vi "KM101_SetChannelZero.vi"(9 "Channel":i32, 10 "reference in":refnum<k7>) -> (2 "reference out":refnum<k7>)   [LabVIEW 2018, in "KIM101lib.lvlib"]
uses:
  KIM101lib.lvlib
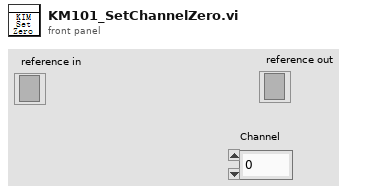
[diagram p1: front panel]
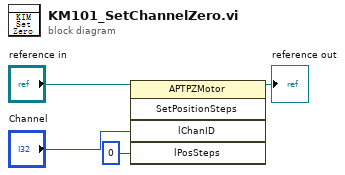
[diagram p0: block diagram]
diagram:
  n1 = invoke class="APTPZMotor" method="SetPositionSteps"(reference="reference in", "lChanID"="Channel", "lPosSteps"=0) -> (reference out=→"reference out":refnum<k7>)  [unwired: 2 in, 4 out]
